vi "运维调试_总磷氨氮.vi"() -> ()   [LabVIEW 2016, in "斯坦道仪器.lvlib"]
uses:
  <vilib>/Platform/TimedLoop/XDataNode/timing_clust.ctl
  <vilib>/Platform/TimedLoop/XDataNode/nitl_modes.ctl
  <vilib>/Platform/TimedLoop/XDataNode/wakeup.ctl
  <vilib>/Utility/miscctls.llb/LVPointTypeDef.ctl
  <vilib>/Platform/TimedLoop/XDataNode/XDataNode.xnode
  <vilib>/Platform/TimedLoop/XDataNode/XDNodeRunTimeDep.lvlib
panel:
  out "固件版本号":string
  in  "参数":T1={"站号"=1, "量程切换"=enum."AUTO", "控制命令"=enum."启动测量", "模式设置"=enum."待机", "测量间隔"=0} {"站号" items=["总磷"=1, "氨氮"=3]}
  out "error out":errorcluster
  in  "同步时间":bool
  in  "数组":string[](array[string])
  in  "备用系数写入":bool
  in  "备用系数读取":bool
  in  "备用系数":T2
  in  "量程切换阈值写入":bool
  in  "量程切换阈值读取":bool
  in  "量程切换阈值":cluster{"阈值":dbl, "标液浓度":dbl}
  in  "参数下拉列表":enum16{"氨氮", "总磷"}(ring)
  in  "量程下拉列表":enum16{"低量程", "高量程"}(ring)
  in  "测量模式下拉列表":enum16{"水样测量", "空白核查", "标样核查", "盲样测试", "加标回收"}(ring)
  in  "公式":cluster{"X^2":dbl, "X":dbl, "b":dbl}
  in  "写公式":bool
  in  "读公式":bool
  in  "精度":dbl=4.0
  in  "样品5 F0":dbl
  in  "样品5 F1":dbl
  in  "样品4 F1":dbl
  in  "样品4 F0":dbl
  in  "样品3 F0":dbl
  in  "样品3 F1":dbl
  in  "样品2 F0":dbl
  in  "样品2 F1":dbl
  in  "样品1 F1":dbl
  in  "样品1 F0":dbl
  in  "method":u16(ring) items=["最小二乘", "最小绝对残差", "Bisquare"]
  in  "模型":enum32{"线性", "多项式"}(ring)
  out "r^2":dbl format="%.7g"
  out "拟合公式":string
  in  "样品2启用":bool
  in  "样品5启用":bool
  in  "样品4启用":bool
  in  "样品3启用":bool
  in  "样品1启用":bool
  in  "标液浓度5":dbl
  out "测量吸光度5":dbl
  in  "标液浓度4":dbl
  out "测量吸光度4":dbl
  in  "标液浓度3":dbl
  out "测量吸光度3":dbl
  in  "标液浓度2":dbl
  out "测量吸光度2":dbl
  out "测量吸光度1":dbl
  in  "标液浓度1":dbl
  out "XY图":cluster{"X Values":dbl[], "Y Values":dbl[]}[](graph)
  in  "返回":bool
  in  "设置":bool
  out "序列号":string="序列号"
  out "氨氮测量数据":T3(xcontrol)
  out "总磷测量数据":T3(xcontrol)
  out "集成报警信息":string
  out "设置值":dbl
  out "定时启动":bool
  out "总磷总氮运行状态":T4(xcontrol)
  in  "停止":bool
  in  "手动启动":bool
  in  "单步测试":bool
  in  "总磷氨氮调试":u16[](xcontrol)
  out "F3":sgl format="%#.6f"
  out "F2":sgl format="%#.6f"
  out "F1":sgl format="%#.6f"
  out "F0":sgl format="%#.6f"
  out "多列列表框":i32(listbox)
  # "COM4"
  # "参数设置"
  # "标液浓度"
  # "F0"
  # "F1"
  # "吸光值显示"
  # "样品一"
  # "辅\n助\n计\n算\n区"
  # "样品二"
  # "样品三"
  # "样品四"
  # "样品五"
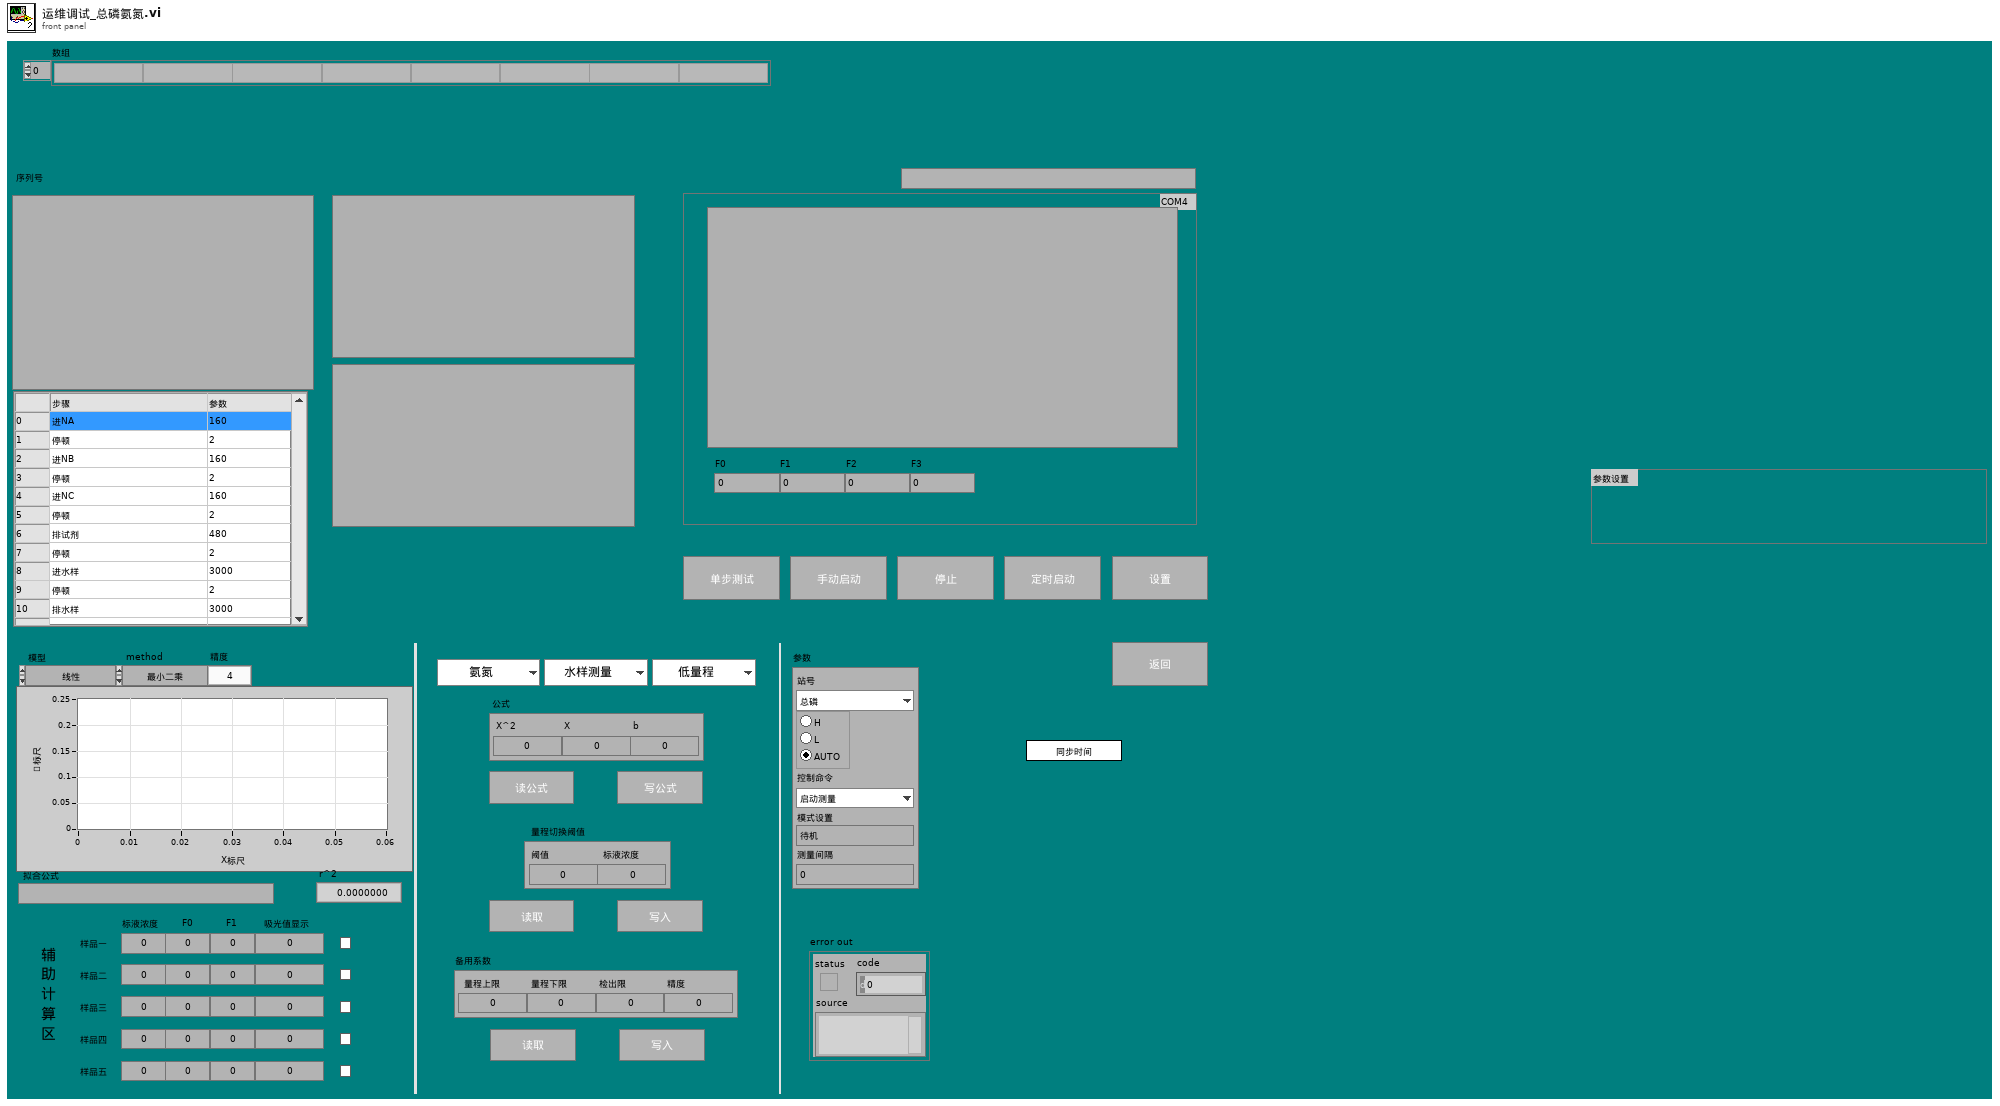
[diagram p1: front panel]
types:
  T1 = cluster{"站号":u16, "量程切换":enum32{"H", "L", "AUTO"}, "控制命令":enum16{"启动测量", "标样核查", "零点核查", "跨度核查", "空白测试", "平行样测试", "加标回收", "空白校准", "标样校准", "初始化（清洗）", "停止测试", "仪器重启", "校时", "模式设置", "测量间隔设置", ""}, "模式设置":enum16{"待机", "连续模式", "周期模式", "定点模式", "受控模式", "手动模式"}, "测量间隔":u16}
  T2 = cluster{"量程上限":dbl, "量程下限":dbl, "检出限":dbl, "精度":dbl}
  T3 = cluster{"flowid":u16, "测量精度":u16, "测量数据区":cluster{"因子编码":u32, "单位":u16, "标样参考值":sgl, "水样数据时间":timestamp, "水样实测值":sgl, "水样数据标识":string, "标样数据时间":timestamp, "标样实测值":sgl, "标样数据标识":string, "空白数据时间":timestamp, "空白实测值":sgl, "空白数据标识":string, "零点核查数据时间":timestamp, "零点核查实测值":sgl, "零点核查数据标识":string, "跨度核查数据时间":timestamp, "跨度核查实测值":sgl, "跨度核查数据标识":string, "加标回收数据时间":timestamp, "加标回收实测值":sgl, "加标回收数据标识":string, "平行样数据时间":timestamp, "平行样实测值":sgl, "平行样数据标识":string}}
  T4 = cluster{"系统时间":timestamp, "工作状态":enum16{"空闲", "水样测试", "标样核查", "零点核查", "跨度核查", "空白测试", "平行样测试", "加标回收", "空白校准", "标样校准", "初始化（清洗）"}, "测量模式":enum16{"待机", "连续模式", "周期模式", "定点模式", "受控模式", "手动模式"}, "告警代码":enum16{"无告警", "缺试剂告警", "缺水样告警", "缺蒸馏水告警", "缺标液告警", "仪表漏液告警", "标定异常告警", "超量程告警", "加热异常", "低试剂预警", "超上限告警", "超下限告警", "仪表内部其他异常", "滴定异常告警", "电极异常告警", "量程切换告警", "参数设置告警", "PH电极电位异常", "电导率电极异常", "浊度光度异常", "溶解氧电极异常", "溶解氧光强异常", "温度异常告警", "PH异常告警", "溶解氧异常告警", "电导率异常告警", "浊度异常告警", "叶绿素异常告警", "藻密度异常告警", "蓝绿藻异常告警", "ORP异常告警", "氨氮异常告警", "清洁刷异常告警", "SD卡异常告警", "蓝牙异常告警", "Wifi异常告警", "流程异常告警"}, "故障代码":enum16{"无故障", "电机故障", "温度故障", "通讯故障", "滴定故障"}, "日志代码":u16, "软件版本":u16, "F0":sgl, "F1":sgl, "F2":sgl, "F3":sgl, "T":sgl, "H":sgl, "id":u16, "flowid":u16, "量程":u16}
  T5 = enum16{"待机", "启动氨氮", "氨氮测量中", "启动总磷", "总磷测量中", "延时"}
  T6 = typedef "LVPointTypeDef.ctl" = cluster{"Horizontal":i16, "Vertical":i16}
  T7 = cluster{"因子编码":u32, "单位":u16, "标样参考值":sgl, "水样数据时间":timestamp, "水样实测值":sgl, "水样数据标识":string, "标样数据时间":timestamp, "标样实测值":sgl, "标样数据标识":string, "空白数据时间":timestamp, "空白实测值":sgl, "空白数据标识":string, "零点核查数据时间":timestamp, "零点核查实测值":sgl, "零点核查数据标识":string, "跨度核查数据时间":timestamp, "跨度核查实测值":sgl, "跨度核查数据标识":string, "加标回收数据时间":timestamp, "加标回收实测值":sgl, "加标回收数据标识":string, "平行样数据时间":timestamp, "平行样实测值":sgl, "平行样数据标识":string}
  T8 = enum16{"空闲", "水样测试", "标样核查", "零点核查", "跨度核查", "空白测试", "平行样测试", "加标回收", "空白校准", "标样校准", "初始化（清洗）"}
  T9 = cluster{"启动模式":enum16{"标液测量", "水样测量", "零液测量", "盲样测量", "加标回收"}, "启动参数":u16, "量程":enum16{"低量程", "高量程"}}
  T10 = cluster{"时间标识":timestamp, "设备":string, "日志信息":string, "流程参数":string}
  T11 = cluster{"时间标识":timestamp, "设备":string, "日志信息":string}
  T12 = enum16{"无告警", "缺试剂告警", "缺水样告警", "缺蒸馏水告警", "缺标液告警", "仪表漏液告警", "标定异常告警", "超量程告警", "加热异常", "低试剂预警", "超上限告警", "超下限告警", "仪表内部其他异常", "滴定异常告警", "电极异常告警", "量程切换告警", "参数设置告警", "PH电极电位异常", "电导率电极异常", "浊度光度异常", "溶解氧电极异常", "溶解氧光强异常", "温度异常告警", "PH异常告警", "溶解氧异常告警", "电导率异常告警", "浊度异常告警", "叶绿素异常告警", "藻密度异常告警", "蓝绿藻异常告警", "ORP异常告警", "氨氮异常告警", "清洁刷异常告警", "SD卡异常告警", "蓝牙异常告警", "Wifi异常告警", "流程异常告警"}
  T13 = typedef "LVRowAndColumnUnsignedTypeDef.ctl" = cluster{"Row":u32, "Column":u32}
  T14 = typedef "XDNodeRunTimeDep.lvlib/timing_clust.ctl" = cluster{"Expected End [f-1]":u64, "Actual End [f-1]":u64, "Finished Late? [f-1]":bool, "Expected End [i-1]":u64, "Actual End [i-1]":u64, "Finished Late? [i-1]":bool, "Expected Start [i]":u64, "Actual Start [i]":u64, "Expected Start [f]":u64, "Actual Start [f]":u64, "Source Name":string, "Structure Name":string, "Period":i64, "Deadline":i64, "Offset":i64, "Start":i64, "Priority":i32, "Timeout":i32, "Mode":T15, "Wakeup Reason":T16, "Error":errorcluster, "Source Type":string, "Secondary Source Type":string, "Global End Time":u64, "Global Start Time":u64, "Frame Duration":u64, "Iteration Duration":u64, "Assigned CPU":i32, "I/O Scan Engine Mode":u32}
  T15 = typedef "XDNodeRunTimeDep.lvlib/nitl_modes.ctl" = enum32{"No Change", "Process missed periods, maintain original phase", "Discard missed periods, maintain original phase", "Process missed periods, ignore original phase", "Discard missed periods, ignore original phase"}
  T16 = typedef "XDNodeRunTimeDep.lvlib/wakeup.ctl" = enum32{"Normal", "Aborted", "Asynchronous wakeup", "Timing source error", "Timed loop error", "Timeout"}
  T17 = cluster{"站号":u16, "量程切换":enum32{"H", "L", "AUTO"}, "控制命令":enum16{"启动测量", "标样核查", "零点核查", "跨度核查", "空白测试", "平行样测试", "加标回收", "空白校准", "标样校准", "初始化（清洗）", "停止测试", "仪器重启", "校时", "模式设置", "测量间隔设置", "盲样测试"}, "模式设置":enum16{"待机", "连续模式", "周期模式", "定点模式", "受控模式", "手动模式"}, "测量间隔":u16}
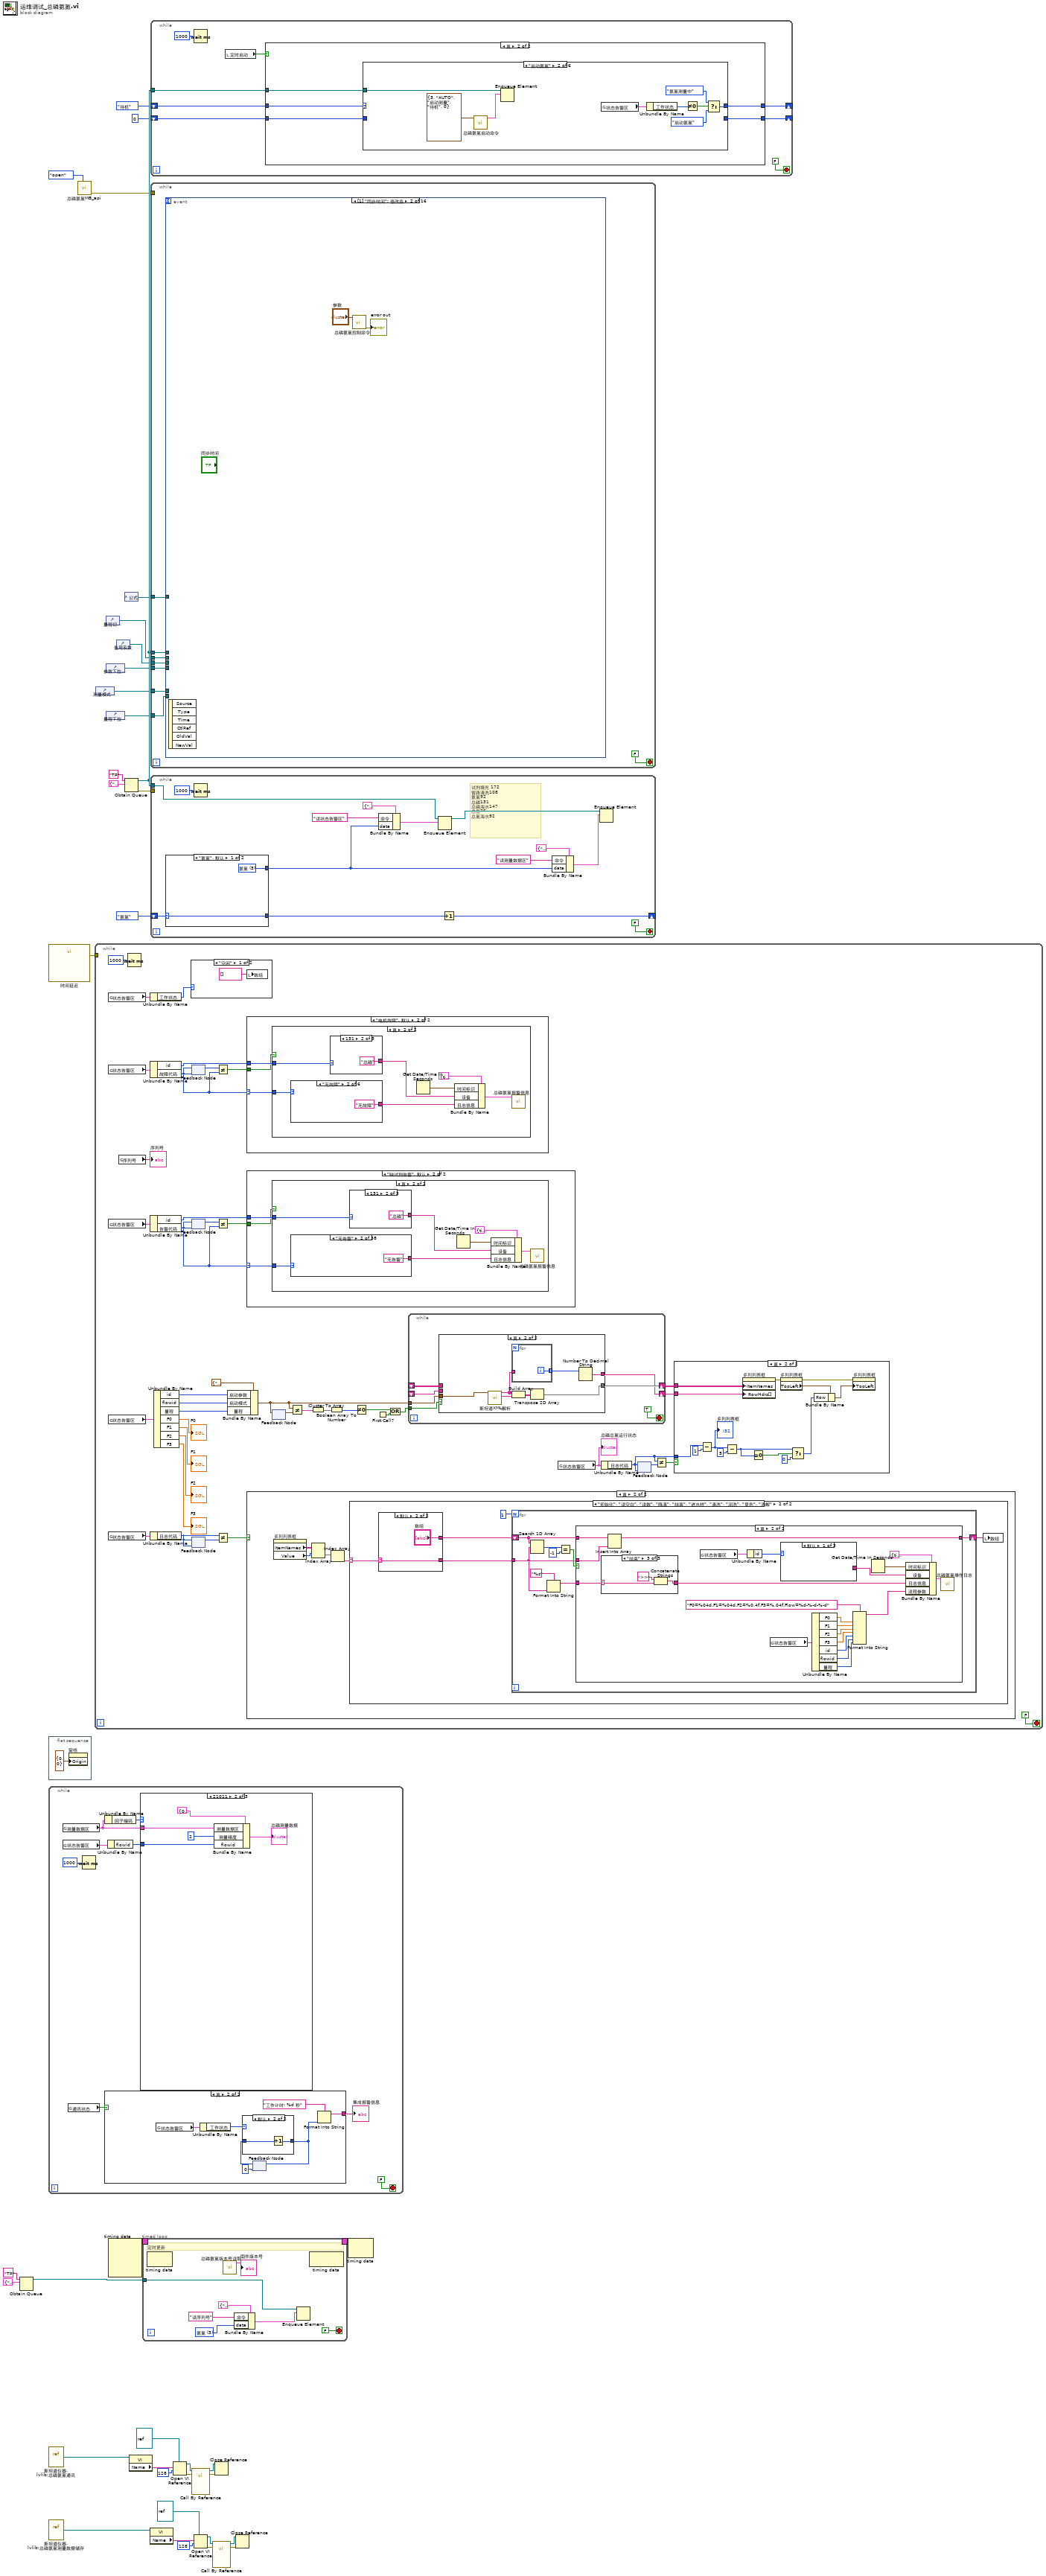
[diagram p0: block diagram]
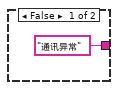
[diagram p2: hidden frame]
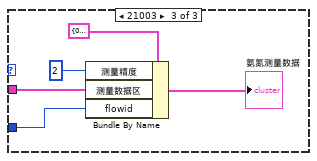
[diagram p5: hidden frame]
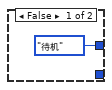
[diagram p6: hidden frame]
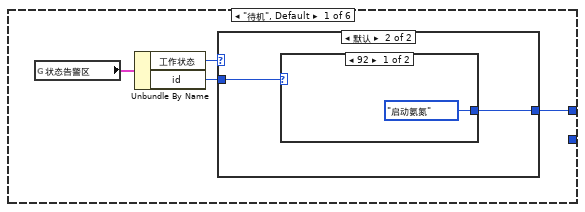
[diagram p7: hidden frame]
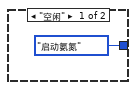
[diagram p8: hidden frame]
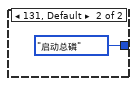
[diagram p9: hidden frame]
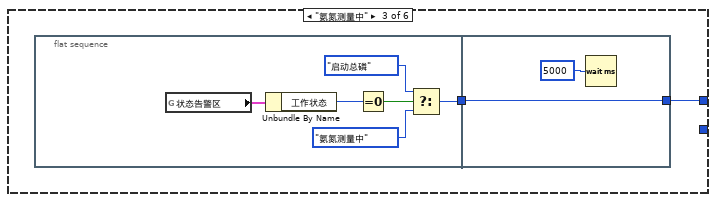
[diagram p10: hidden frame]
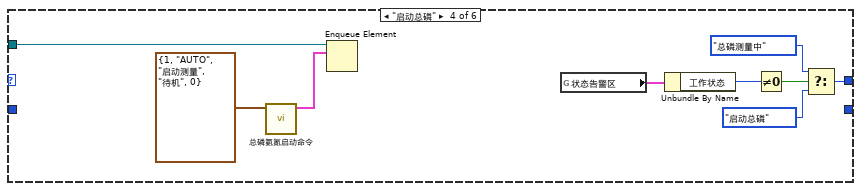
[diagram p11: hidden frame]
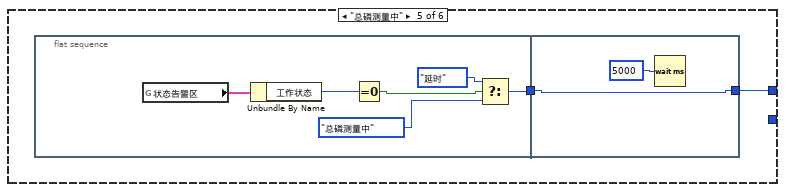
[diagram p12: hidden frame]
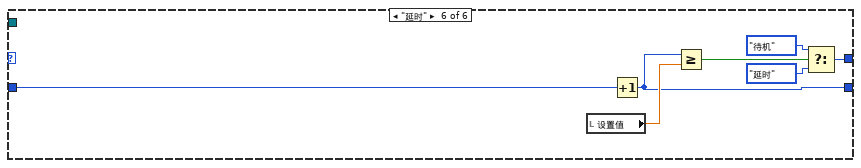
[diagram p13: hidden frame]
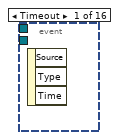
[diagram p14: hidden frame]
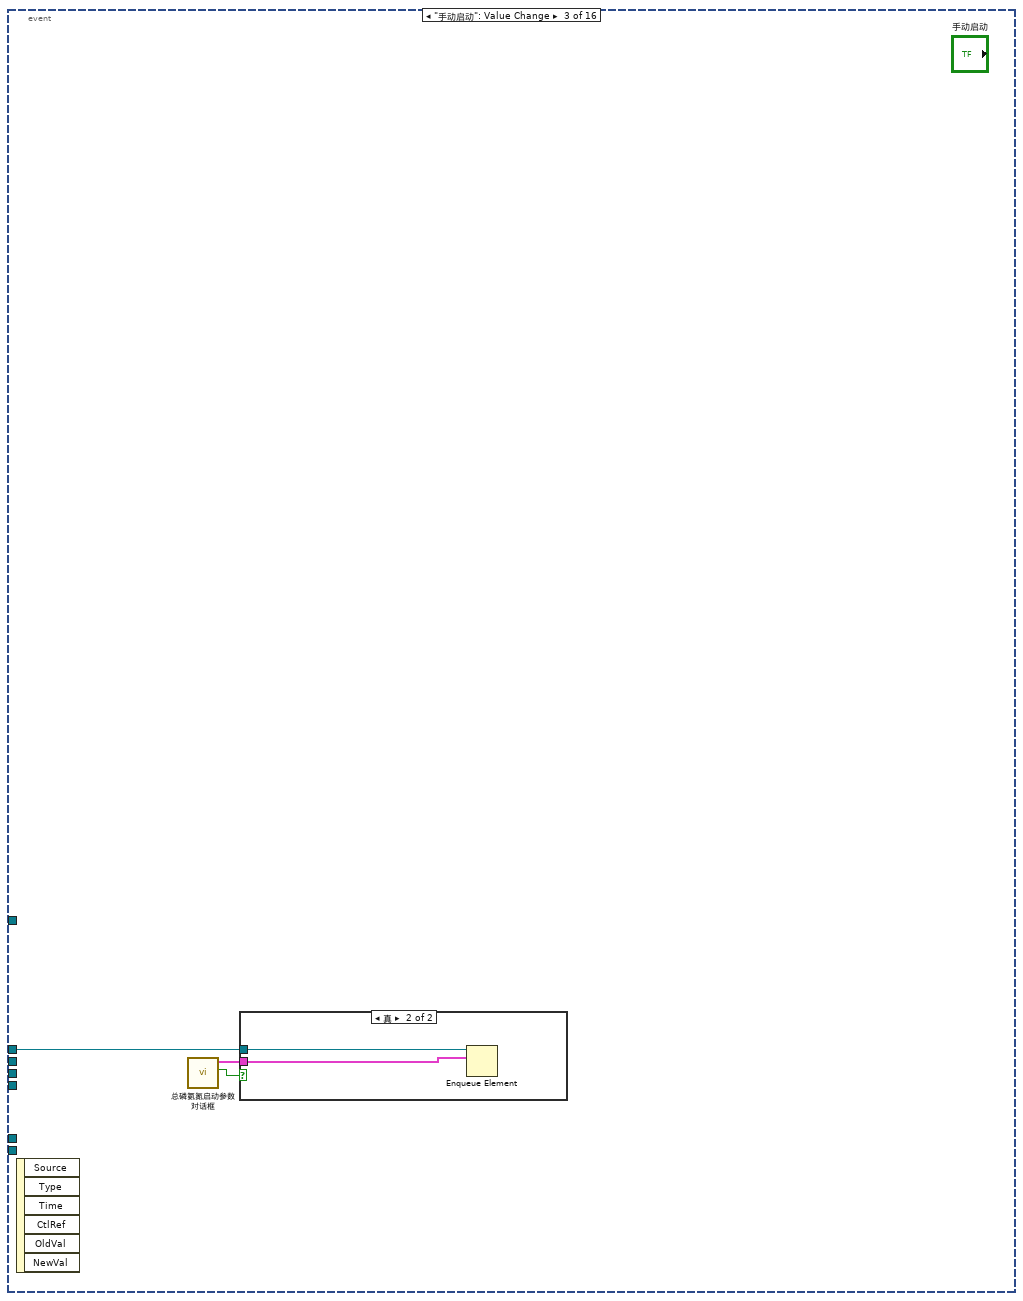
[diagram p15: hidden frame]
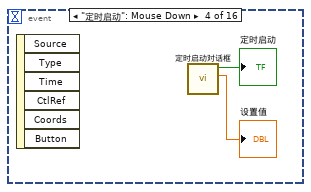
[diagram p17: hidden frame]
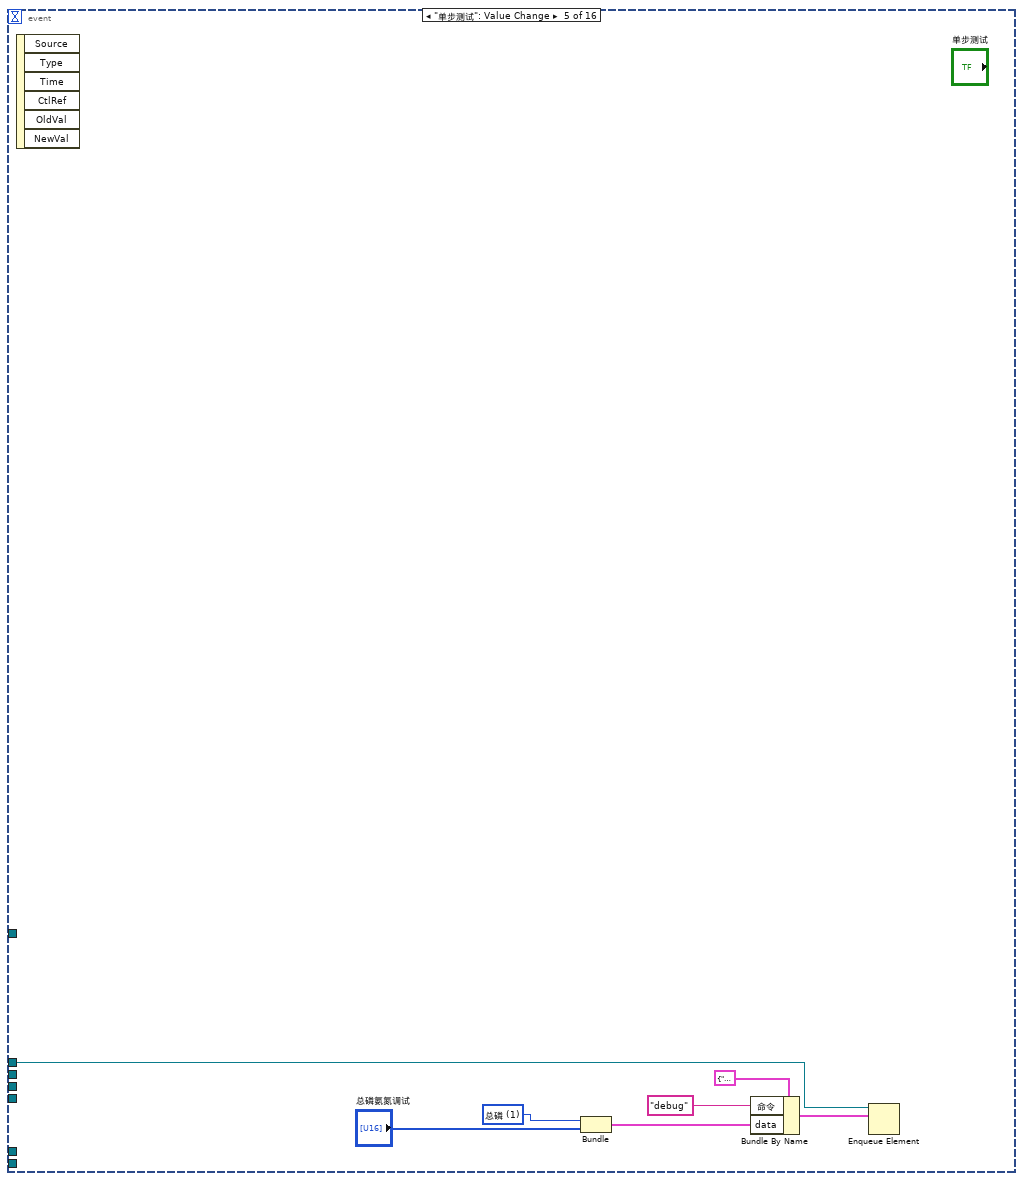
[diagram p18: hidden frame]
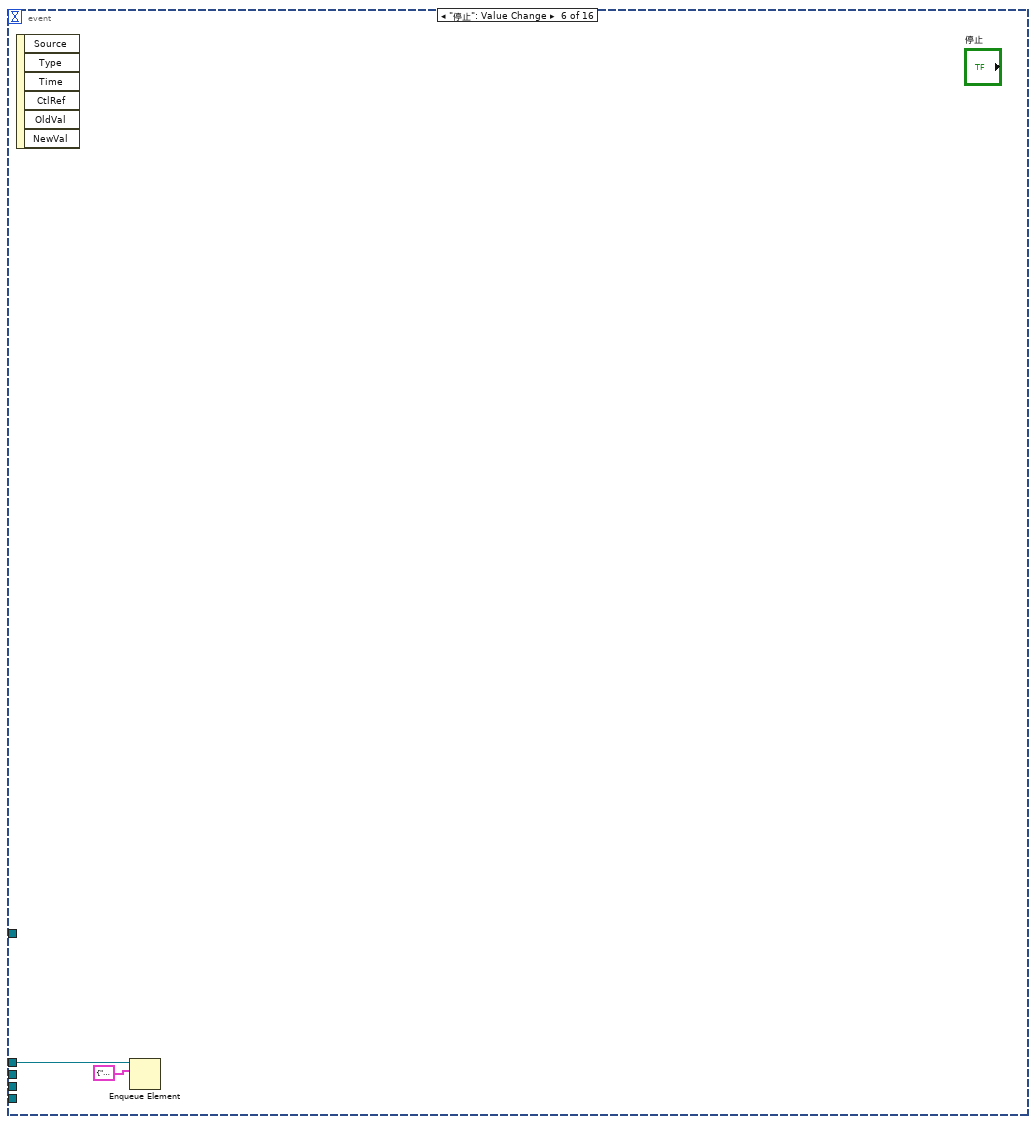
[diagram p19: hidden frame]
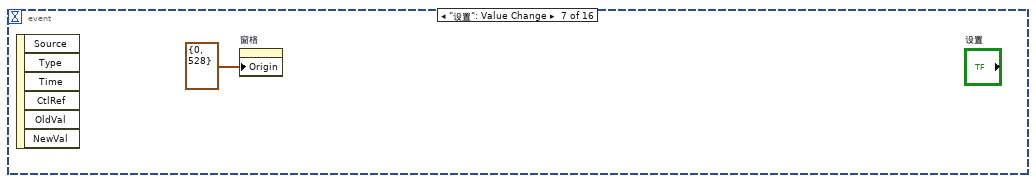
[diagram p20: hidden frame]
diagram:
  n1 = Obtain Queue(name (unnamed)="TP" ("名称（未命名）"), element data type=cluster{"命令":string, "data":variant} {"命令"="", "data"=variant}) -> (queue out=w1:refnum<queue>)  [unwired: 3 in, 2 out]
  n2 = call "时间延迟"() -> ("error out"=w8:errorcluster)  [unwired: 11 in]
  n3 = flat-sequence {
    frame #0 {
      n4 = property on="窗格" class="Pane"("Origin"=T6 {"Horizontal"=0, "Vertical"=0} ("原点")) -> ()  [unwired: 2 in, 2 out]
    }
  }
  n5 = while {
    stop <- FALSE stop-if-true
    n6 = global read "VAR总磷氨氮全局变量.vi" "测量数据区"() -> (w44:T7)
    n7 = global read "VAR总磷氨氮全局变量.vi" "状态告警区"() -> (w40:T4)
    n8 = global read "VAR总磷氨氮全局变量.vi" "通讯状态"() -> (w42:bool)
    n9 = Wait (ms)(milliseconds to wait=u32 1000 ("等待时间（毫秒）")) -> ()  [unwired: 1 out]
    n10 = Unbundle By Name(w44) -> ("因子编码"=w43:u32)
    n11 = case shown="真" w42 {
      tunnel: ["通讯异常" ("集成报警信息") w48] -> w41
      frame False {
      }
      frame True {
        n12 = global read "VAR总磷氨氮全局变量.vi" "状态告警区"() -> (w54:T4)
        n13 = Unbundle By Name(w54) -> ("工作状态"=w53:T8)
        n14 = feedback #1(0) -> (w51:i32)
        n15 = case shown="默认" w53 {
          tunnel: w51 -> [_ w56]
          tunnel: [_ w55] -> w49
          frame "空闲" {
          }
          frame Default {
            n16 = Increment(x=w56) -> (x+1=w55:i32)
          }
        }
        n17 = feedback-in #1(w49) -> ()
        n18 = Format Into String(format string="工作计时: %d 秒" ("格式字符串"), w49) -> (resulting string=w48:string)  [unwired: 2 in, 1 out]
      }
    }
    "集成报警信息" <- w41
    n19 = Unbundle By Name(w40) -> ("flowid"=w39:u16)
    n20 = case shown="21011" w43 {
      tunnel: w44 -> [_ w61 w66]
      tunnel: w39 -> [_ w58 w64]
      frame Default {
      }
      frame 21011 {
        n21 = Bundle By Name(cluster=T3 {"flowid"=0, "测量精度"=0, "测量数据区"={"因子编码"=0, "单位"=0, "标样参考值"=0.0, "水样数据时间"=timestamp(0 s since 1904-01-01), "水样实测值"=0.0, "水样数据标识"="", "标样数据时间"=timestamp(0 s since 1904-01-01), "标样实测值"=0.0, "标样数据标识"="", "空白数据时间"=timestamp(0 s since 1904-01-01), "空白实测值"=0.0, "空白数据标识"="", "零点核查数据时间"=timestamp(0 s since 1904-01-01), "零点核查实测值"=0.0, "零点核查数据标识"="", "跨度核查数据时间"=timestamp(0 s since 1904-01-01), "跨度核查实测值"=0.0, "跨度核查数据标识"="", "加标回收数据时间"=timestamp(0 s since 1904-01-01), "加标回收实测值"=0.0, "加标回收数据标识"="", "平行样数据时间"=timestamp(0 s since 1904-01-01), "平行样实测值"=0.0, "平行样数据标识"=""}} ("氨氮测量数据"), "测量数据区"=w61, "测量精度"=u16 2, "flowid"=w58) -> (→"总磷测量数据":T3)
      }
      frame 21003 {
        n22 = Bundle By Name(cluster=T3 {"flowid"=0, "测量精度"=0, "测量数据区"={"因子编码"=0, "单位"=0, "标样参考值"=0.0, "水样数据时间"=timestamp(0 s since 1904-01-01), "水样实测值"=0.0, "水样数据标识"="", "标样数据时间"=timestamp(0 s since 1904-01-01), "标样实测值"=0.0, "标样数据标识"="", "空白数据时间"=timestamp(0 s since 1904-01-01), "空白实测值"=0.0, "空白数据标识"="", "零点核查数据时间"=timestamp(0 s since 1904-01-01), "零点核查实测值"=0.0, "零点核查数据标识"="", "跨度核查数据时间"=timestamp(0 s since 1904-01-01), "跨度核查实测值"=0.0, "跨度核查数据标识"="", "加标回收数据时间"=timestamp(0 s since 1904-01-01), "加标回收实测值"=0.0, "加标回收数据标识"="", "平行样数据时间"=timestamp(0 s since 1904-01-01), "平行样实测值"=0.0, "平行样数据标识"=""}} ("氨氮测量数据"), "测量精度"=u16 2, "测量数据区"=w66, "flowid"=w64) -> (→"氨氮测量数据":T3)
      }
    }
  }
  n23 = vi-ref "斯坦道仪器.lvlib:总磷氨氮通讯.vi"() -> (w31:refnum<vi>)
  n24 = vi-ref "斯坦道仪器.lvlib:总磷氨氮测量数据储存.vi"() -> (w23:refnum<vi>)
  n25 = call "总磷氨氮MB_api.vi"("STEP"=enum16{"open", "read", "write", "close"}."open") -> ("error out"=w7:errorcluster)  [unwired: 8 in, 2 out]
  n26 = while {
    tunnel: w8 -> [_]
    stop <- FALSE stop-if-true
    n27 = global read "VAR总磷氨氮全局变量.vi" "状态告警区"() -> (w72:T4)
    n28 = global read "VAR总磷氨氮全局变量.vi" "状态告警区"() -> (w78:T4)
    n29 = global read "VAR总磷氨氮全局变量.vi" "状态告警区"() -> (w83:T4)
    n30 = global read "VAR总磷氨氮全局变量.vi" "状态告警区"() -> (w95:T4)
    n31 = global read "VAR总磷氨氮全局变量.vi" "状态告警区"() -> (w69:T4)
    n32 = global read "VAR总磷氨氮全局变量.vi" "序列号"() -> (→"序列号":string)
    n33 = Wait (ms)(milliseconds to wait=u32 1000 ("等待时间（毫秒）")) -> ()  [unwired: 1 out]
    n34 = Unbundle By Name(w72) -> ("工作状态"=w71:T8)
    n35 = Unbundle By Name(w78) -> ("id"=w77:u16, "故障代码"=w74:enum16{"无故障", "电机故障", "温度故障", "通讯故障", "滴定故障"})
    n36 = Unbundle By Name(w83) -> ("id"=w82:u16, "告警代码"=w79:T12)
    n37 = Unbundle By Name(w69) -> ("日志代码"=w68:u16)
    n38 = Unbundle By Name(w95) -> ("id"=w92:u16, "flowid"=w94:u16, "量程"=w93:u16, "F0"=→"F0":sgl, "F1"=→"F1":sgl, "F2"=→"F2":sgl, "F3"=→"F3":sgl)
    n39 = case shown="\"空闲\"" w71 {
      frame "空闲" {
        n40 = local write "数组"(string[] [] ("数组")) -> ()
      }
      frame "水样测试", Default {
      }
    }
    n41 = feedback #2(w74) -> (w75:enum16{"无故障", "电机故障", "温度故障", "通讯故障", "滴定故障"})
    n42 = feedback-in #2(w74) -> ()
    n43 = feedback #3(w79) -> (w80:T12)
    n44 = feedback-in #3(w79) -> ()
    n45 = feedback #4(w68) -> (w70:u16)
    n46 = feedback-in #4(w68) -> ()
    n47 = Not Equal?(x=w75, y=w74) -> (x != y?=w76:bool)
    n48 = Not Equal?(x=w80, y=w79) -> (x != y?=w81:bool)
    n49 = Not Equal?(x=w68, y=w70) -> (x != y?=w67:bool)
    n50 = Bundle By Name(cluster=T9 {"启动模式"=enum."加标回收", "启动参数"=1, "量程"=enum."低量程"} ("参数簇"), "启动参数"=w92, "启动模式"=w94, "量程"=w93) -> (w85:T9)
    n51 = case shown="\"电机故障\", 默认" w74 {
      selector: w74 -> [_ w163]
      tunnel: w77 -> [_ w164]
      tunnel: w76 -> [_ w162]
      frame "无故障" {
      }
      frame "电机故障", Default {
        n52 = case shown="真" w162 {
          tunnel: w164 -> [_ w171]
          tunnel: w163 -> [_ w166]
          frame False {
          }
          frame True {
            n53 = case shown="\"无故障\"" w166 {
              selector: w166 -> [w173 _ _ _ _ _]
              tunnel: [w172 "无故障" "电机故障" "温度故障" "通讯故障" "滴定故障"] -> w165
              frame Default {
                n54 = Format Into String(format string="%d" ("格式字符串"), initial string="未知" ("工作状态"), w173) -> (resulting string=w172:string)  [unwired: 1 in, 1 out]
              }
              frame "无故障" {
              }
              frame "电机故障" {
              }
              frame "温度故障" {
              }
              frame "通讯故障" {
              }
              frame "滴定故障" {
              }
            }
            n55 = case shown="131" w171 {
              tunnel: [_ "总磷" ("table输入") "氨氮" ("table输入")] -> w167
              frame Default {
              }
              frame 131 {
              }
              frame 92 {
              }
            }
            n56 = Get Date/Time In Seconds() -> (seconds since 1Jan1904=w168:timestamp)
            n57 = Bundle By Name(cluster=T11 {"时间标识"=timestamp(0 s since 1904-01-01), "设备"="", "日志信息"=""} ("data in"), "时间标识"=w168, "设备"=w167, "日志信息"=w165) -> (w169:T11)
            n58 = call "总磷氨氮报警信息.vi"("data in"=w169) -> ()  [unwired: 11 in]
          }
        }
      }
    }
    n59 = case shown="\"缺试剂告警\", 默认" w79 {
      selector: w79 -> [_ w184]
      tunnel: w82 -> [_ w185]
      tunnel: w81 -> [_ w183]
      frame "无告警" {
      }
      frame "缺试剂告警", Default {
        n60 = case shown="真" w183 {
          tunnel: w185 -> [_ w192]
          tunnel: w184 -> [_ w186]
          frame False {
          }
          frame True {
            n61 = case shown="\"无告警\"" w186 {
              selector: w186 -> [w194 _ _ _ _ _ _ _ _ _ _ _ _ _ _ _ _ _ _ _ _ _ _ _ _ _ _ _ _ _ _ _ _ _ _ _ _ _]
              tunnel: [w193 "无告警" "缺试剂告警" "缺水样告警" "缺蒸馏水告警" "缺标液告警" "仪表漏液告警" "标定异常告警" "超量程告警" "加热异常" "低试剂预警" "超上限告警" "超下限告警" "仪表内部其他异常" "滴定异常告警" "电极异常告警" "量程切换告警" "参数设置告警" "PH电极电位异常" "电导率电极异常" "浊度光度异常" "溶解氧电极异常" "溶解氧光强异常" "温度异常告警" "PH异常告警" "溶解氧异常告警" "电导率异常告警" "浊度异常告警" "叶绿素异常告警" "藻密度异常告警" "蓝绿藻异常告警" "ORP异常告警" "氨氮异常告警" "清洁刷异常告警" "SD卡异常告警" "蓝牙异常告警" "WiFi异常告警" "流程异常告警"] -> w187
              frame Default {
                n62 = Format Into String(format string="%d" ("格式字符串"), initial string="未知" ("工作状态"), w194) -> (resulting string=w193:string)  [unwired: 1 in, 1 out]
              }
              frame "无告警" {
              }
              frame "缺试剂告警" {
              }
              frame "缺水样告警" {
              }
              frame "缺蒸馏水告警" {
              }
              frame "缺标液告警" {
              }
              frame "仪表漏液告警" {
              }
              frame "标定异常告警" {
              }
              frame "超量程告警" {
              }
              frame "加热异常" {
              }
              frame "低试剂预警" {
              }
              frame "超上限告警" {
              }
              frame "超下限告警" {
              }
              frame "仪表内部其他异常" {
              }
              frame "滴定异常告警" {
              }
              frame "电极异常告警" {
              }
              frame "量程切换告警" {
              }
              frame "参数设置告警" {
              }
              frame "PH电极电位异常" {
              }
              frame "电导率电极异常" {
              }
              frame "浊度光度异常" {
              }
              frame "溶解氧电极异常" {
              }
              frame "溶解氧光强异常" {
              }
              frame "温度异常告警" {
              }
              frame "PH异常告警" {
              }
              frame "溶解氧异常告警" {
              }
              frame "电导率异常告警" {
              }
              frame "浊度异常告警" {
              }
              frame "叶绿素异常告警" {
              }
              frame "藻密度异常告警" {
              }
              frame "蓝绿藻异常告警" {
              }
              frame "ORP异常告警" {
              }
              frame "氨氮异常告警" {
              }
              frame "清洁刷异常告警" {
              }
              frame "SD卡异常告警" {
              }
              frame "蓝牙异常告警" {
              }
              frame "Wifi异常告警" {
              }
              frame "流程异常告警" {
              }
            }
            n63 = case shown="131" w192 {
              tunnel: [_ "总磷" ("table输入") "氨氮" ("table输入")] -> w188
              frame Default {
              }
              frame 131 {
              }
              frame 92 {
              }
            }
            n64 = Get Date/Time In Seconds() -> (seconds since 1Jan1904=w189:timestamp)
            n65 = Bundle By Name(cluster=T11 {"时间标识"=timestamp(0 s since 1904-01-01), "设备"="", "日志信息"=""} ("data in"), "时间标识"=w189, "设备"=w188, "日志信息"=w187) -> (w190:T11)
            n66 = call "总磷氨氮报警信息.vi"("data in"=w190) -> ()  [unwired: 11 in]
          }
        }
      }
    }
    n67 = case shown="真" w67 {
      frame False {
      }
      frame True {
        n68 = property on="多列列表框" class="MCListbox (严格)"() -> ("ItemNames"=w112:string[][], "Value"=w113:i32)  [unwired: 2 in, 2 out]
        n69 = Index Array(array=w112, index (row)=w113) -> (element=w111:string[])  [unwired: 1 in]
        n70 = Index Array(array=w111) -> (element=w110:string)  [unwired: 1 in]
        n71 = case shown="\"初始化\", \"读空白\", \"读数\", \"降温\", \"结束\", \"进水样\", \"清洗\", \"润洗\", \"显色\", \"消解\"" w110 {
          selector: w110 -> [_ w116]
          frame Default {
          }
          frame "初始化", "读空白", "读数", "降温", "结束", "进水样", "清洗", "润洗", "显色", "消解" {
            n72 = case shown="默认" w116 {
              selector: w116 -> [w120 w122]
              tunnel: [w120 w122] -> w115
              tunnel: [string[] [] ("数组") "数组"] -> w114
              frame "读数" {
              }
              frame Default {
              }
            }
            n73 = for {
              N: 1 -> [_]
              tunnel: w115 -> [w124]
              shift-right: [w123] -> w117
              shift-left: w114 -> [w125]
              n74 = Search 1D Array(1D array=w125, element=w124) -> (index of element=w128:i32)  [unwired: 1 in]
              n75 = Format Into String(format string="%s" ("格式字符串"), w124) -> (resulting string=w129:string)  [unwired: 2 in, 1 out]
              n76 = Equal?(x=w128, y=-1) -> (x = y?=w126:bool)
              n77 = case shown="真" w126 {
                tunnel: w129 -> [_ w133]
                tunnel: w125 -> [w131 w137]
                tunnel: w124 -> [_ w136]
                tunnel: [w131 w135] -> w123
                frame False {
                }
                frame True {
                  n78 = case shown="\"结束\"" w133 {
                    selector: w133 -> [w153 w156 w159]
                    tunnel: [w153 w155 w158] -> w132
                    frame Default {
                    }
                    frame "初始化" {
                      n79 = Concatenate Strings("<<" ("字符串"), w156) -> (w155:string)
                    }
                    frame "结束" {
                      n80 = Concatenate Strings(">>" ("字符串"), w159) -> (w158:string)
                    }
                  }
                  n81 = Insert Into Array(array=w137, new element=w136) -> (w135:string[])  [unwired: 1 in]
                  n82 = global read "VAR总磷氨氮全局变量.vi" "状态告警区"() -> (w152:T4)
                  n83 = Unbundle By Name(w152) -> ("id"=w151:u16)
                  n84 = global read "VAR总磷氨氮全局变量.vi" "状态告警区"() -> (w147:T4)
                  n85 = case shown="默认" w151 {
                    tunnel: [_ "总磷" ("table输入") "氨氮" ("table输入")] -> w149
                    frame Default {
                    }
                    frame 131 {
                    }
                    frame 92 {
                    }
                  }
                  n86 = Unbundle By Name(w147) -> ("F0"=w144:sgl, "F1"=w143:sgl, "F2"=w142:sgl, "F3"=w141:sgl, "id"=w140:u16, "flowid"=w139:u16, "量程"=w138:u16)
                  n87 = Format Into String(format string="F0=%04d,F1=%04d,F2=%0.4f,F3=%.04f,Flow=%d-%-d-%-d" ("格式字符串"), w144, w143, w142, w141, w140, w139, w138) -> (resulting string=w145:string)  [unwired: 2 in, 1 out]
                  n88 = Get Date/Time In Seconds() -> (seconds since 1Jan1904=w148:timestamp)
                  n89 = Bundle By Name(cluster=T10 {"时间标识"=timestamp(0 s since 1904-01-01), "设备"="", "日志信息"="", "流程参数"=""} ("data in"), "时间标识"=w148, "设备"=w149, "日志信息"=w132, "流程参数"=w145) -> (w150:T10)
                  n90 = call "总磷氨氮操作日志.vi"("data in"=w150) -> ()  [unwired: 11 in]
                }
              }
            }
            n91 = local write "数组"(w117) -> ()
          }
        }
      }
    }
    n92 = feedback #5() -> (w101:T9)  [unwired: 1 in]
    n93 = feedback-in #5(w85) -> ()
    n94 = Not Equal?(x=w85, y=w101) -> (x != y?=w102:cluster{"启动模式":bool, "启动参数":bool, "量程":bool})
    n95 = Cluster To Array(cluster=w102) -> (array=w103:bool[])
    n96 = Boolean Array To Number(Boolean array=w103) -> (number=w104:u32)
    n97 = Not Equal To 0?(x=w104) -> (x != 0?=w97:bool)
    n98 = First Call?() -> (First Call?: T/F=w98:bool)
    n99 = Or(x=w97, y=w98) -> (x .or. y?=w96:bool)
    n100 = while {
      tunnel: w96 -> [w242]
      tunnel: w85 -> [w241]
      shift-right: [w240] -> w100
      shift-left: _ -> [w236]
      shift-right: [w239] -> w99
      shift-left: _ -> [w237]
      stop <- TRUE stop-if-true
      n101 = case shown="真" w242 {
        tunnel: [w244 w251] -> w239
        tunnel: [w243 w250] -> w240
        tunnel: w241 -> [_ w245]
        tunnel: w237 -> [w244 _]
        tunnel: w236 -> [w243 _]
        frame False {
        }
        frame True {
          n102 = call "斯坦道XML解析.vi"("参数簇"=w245) -> ("步骤时间"=w246:string[], "步骤名"=w248:string[])  [unwired: 9 in]
          n103 = for {
            tunnel: w248 -> [_] mode=indexing
            tunnel: [w252] -> w249 mode=indexing
            i -> [w252]
          }
          n104 = Build Array(w248, w246) -> (w247:string[][])
          n105 = Transpose 2D Array(2D array=w247) -> (transposed array=w250:string[][])
          n106 = Number To Decimal String(number=w249) -> (decimal integer string=w251:string[])  [unwired: 1 in]
        }
      }
    }
    n107 = global read "VAR总磷氨氮全局变量.vi" "状态告警区"() -> (w86:T4)
    "总磷总氮运行状态" <- w86
    n108 = Unbundle By Name(w86) -> ("日志代码"=w73:u16)
    n109 = feedback-in #6(w73) -> ()
    n110 = feedback #6(w73) -> (w106:u16)
    n111 = Not Equal?(x=w73, y=w106) -> (x != y?=w105:bool)
    n112 = case shown="真" w105 {
      tunnel: w73 -> [_ w255]
      tunnel: w100 -> [_ w262]
      tunnel: w99 -> [_ w261]
      frame False {
      }
      frame True {
        n113 = Subtract(x=w255, y=1) -> (x-y=w253:i32)
        "多列列表框" <- w253
        n114 = Subtract(x=w253, y=5) -> (x-y=w257:i32)
        n115 = property on="多列列表框" class="MCListbox (严格)"("ItemNames"=w262, "RowHdrs[]"=w261) -> (error out=w263:errorcluster)  [unwired: 2 in, 1 out]
        n116 = Greater Or Equal To 0?(x=w257) -> (x >= 0?=w256:bool)
        n117 = property on="多列列表框" class="MCListbox (严格)"(error in=w263) -> (error out=w264:errorcluster, "TopLeft"=w265:T13)  [unwired: 1 in, 1 out]
        n118 = Select(t=w257, s=w256, f=0) -> (s? t:f=w258:i32)
        n119 = Bundle By Name(cluster=w265, "Row"=w258) -> (w266:T13)
        n120 = property on="多列列表框" class="MCListbox (严格)"(error in=w264, "TopLeft"=w266) -> ()  [unwired: 1 in, 2 out]
      }
    }
  }
  n121 = control-ref of="测量模式下拉列表"() -> (w12:refnum<vi>)
  n122 = control-ref of="量程切换阈值"() -> (w10:refnum<vi>)
  n123 = control-ref of="参数下拉列表"() -> (w13:refnum<vi>)
  n124 = control-ref of="量程下拉列表"() -> (w14:refnum<vi>)
  n125 = node-c288() -> (w5:T14)  [unwired: 4 in]
  n126 = control-ref of="备用系数"() -> (w9:refnum<vi>)
  n127 = control-ref of="公式"() -> (w11:refnum<vi>)
  n128 = Obtain Queue(name (unnamed)="TP" ("名称（未命名）"), element data type=cluster{"命令":string, "data":variant} {"命令"="", "data"=variant}) -> (queue out=w34:refnum<queue>, error out=w35:errorcluster)  [unwired: 3 in, 1 out]
  n129 = property class="VI"(reference=w31) -> ("Name"=w30:string)  [unwired: 1 in, 2 out]
  n130 = timed-loop {
    timing: w5 -> [_]
    timing-out: [_] -> w4
    tunnel: w1 -> [w269]
    stop <- FALSE stop-if-true
    w270 = u16 3 items=["总磷"=1, "氨氮"=3] ("站号")
    # "定时更新"
    n131 = node-c288() -> ()  [unwired: 1 in, 1 out]
    n132 = call "总磷氨氮版本号读取.vi"() -> ("固件版本号"=→"固件版本号":string)  [unwired: 11 in]
    n133 = Bundle By Name(cluster=cluster{"命令":string, "data":variant} {"命令"="", "data"=variant} ("元素"), "命令"="读序列号", "data"=w270) -> (w268:cluster{"命令":string, "data":variant})
    n134 = Enqueue Element(queue=w269, element=w268) -> ()  [unwired: 2 in, 3 out]
    n135 = node-c288() -> ()  [unwired: 1 in, 1 out]
  }
  n136 = property class="VI"(reference=w23) -> ("Name"=w16:string)  [unwired: 1 in, 2 out]
  n137 = while {
    tunnel: w34 -> [w278]
    shift-right: [w279] -> _
    shift-left: T5."待机" -> [w280]
    shift-right: [w276] -> _
    shift-left: u32 0 ("等待时间（毫秒）") -> [w277]
    stop <- FALSE stop-if-true
    n138 = Wait (ms)(milliseconds to wait=u32 1000 ("等待时间（毫秒）")) -> ()  [unwired: 1 out]
    n139 = local read "定时启动"() -> (w281:bool)
    n140 = case shown="真" w281 {
      tunnel: w280 -> [_ w289]
      tunnel: [T5."待机" w288] -> w279
      tunnel: w278 -> [_ w287]
      tunnel: w277 -> [_ w286]
      tunnel: [_ w285] -> w276
      frame False {
      }
      frame True {
        n141 = case shown="\"启动氨氮\"" w289 {
          tunnel: [w290 w302 w309 w320 w328 w340] -> w288
          tunnel: w287 -> [_ w307 _ w326 _ _]
          tunnel: w286 -> [_ _ _ _ _ w343]
          tunnel: [_ _ _ _ _ w339] -> w285
          frame "待机", Default {
            n142 = global read "VAR总磷氨氮全局变量.vi" "状态告警区"() -> (w293:T4)
            n143 = Unbundle By Name(w293) -> ("工作状态"=w291:T8, "id"=w292:u16)
            n144 = case shown="默认" w291 {
              tunnel: w292 -> [_ w296]
              tunnel: [T5."启动氨氮" w295] -> w290
              frame "空闲" {
              }
              frame Default {
                n145 = case shown="92" w296 {
                  tunnel: [T5."启动氨氮" T5."启动总磷"] -> w295
                  frame 92 {
                  }
                  frame 131, Default {
                  }
                }
              }
            }
          }
          frame "启动氨氮" {
            n146 = call "总磷氨氮启动命令.vi"("参数"=T17 {"站号"=3, "量程切换"=enum."AUTO", "控制命令"=enum."启动测量", "模式设置"=enum."待机", "测量间隔"=0}) -> ("启动命令"=w300:cluster{"命令":string, "data":variant})  [unwired: 10 in]
            n147 = Enqueue Element(queue=w307, element=w300) -> ()  [unwired: 2 in, 3 out]
            n148 = global read "VAR总磷氨氮全局变量.vi" "状态告警区"() -> (w306:T4)
            n149 = Unbundle By Name(w306) -> ("工作状态"=w305:T8)
            n150 = Not Equal To 0?(x=w305) -> (x != 0?=w304:bool)
            n151 = Select(t=T5."氨氮测量中", s=w304, f=T5."启动氨氮") -> (s? t:f=w302:T5)
          }
          frame "氨氮测量中" {
            n152 = flat-sequence {
              tunnel: [w313] -> w308
              tunnel: [w317] -> w309
              tunnel: w308 -> [w317]
              frame #0 {
                n153 = global read "VAR总磷氨氮全局变量.vi" "状态告警区"() -> (w314:T4)
                n154 = Unbundle By Name(w314) -> ("工作状态"=w315:T8)
                n155 = Equal To 0?(x=w315) -> (x = 0?=w310:bool)
                n156 = Select(t=T5."启动总磷", s=w310, f=T5."氨氮测量中") -> (s? t:f=w313:T5)
              }
              frame #1 {
                n157 = Wait (ms)(milliseconds to wait=u32 5000 ("等待时间（毫秒）")) -> ()  [unwired: 1 out]
              }
            }
          }
          frame "启动总磷" {
            n158 = call "总磷氨氮启动命令.vi"("参数"=T17 {"站号"=1, "量程切换"=enum."AUTO", "控制命令"=enum."启动测量", "模式设置"=enum."待机", "测量间隔"=0}) -> ("启动命令"=w319:cluster{"命令":string, "data":variant})  [unwired: 10 in]
            n159 = Enqueue Element(queue=w326, element=w319) -> ()  [unwired: 2 in, 3 out]
            n160 = global read "VAR总磷氨氮全局变量.vi" "状态告警区"() -> (w321:T4)
            n161 = Unbundle By Name(w321) -> ("工作状态"=w322:T8)
            n162 = Not Equal To 0?(x=w322) -> (x != 0?=w323:bool)
            n163 = Select(t=T5."总磷测量中", s=w323, f=T5."启动总磷") -> (s? t:f=w320:T5)
          }
          frame "总磷测量中" {
            n164 = flat-sequence {
              tunnel: [w330] -> w327
              tunnel: [w336] -> w328
              tunnel: w327 -> [w336]
              frame #0 {
                n165 = global read "VAR总磷氨氮全局变量.vi" "状态告警区"() -> (w333:T4)
                n166 = Unbundle By Name(w333) -> ("工作状态"=w334:T8)
                n167 = Equal To 0?(x=w334) -> (x = 0?=w329:bool)
                n168 = Select(t=T5."延时", s=w329, f=T5."总磷测量中") -> (s? t:f=w330:T5)
              }
              frame #1 {
                n169 = Wait (ms)(milliseconds to wait=u32 5000 ("等待时间（毫秒）")) -> ()  [unwired: 1 out]
              }
            }
          }
          frame "延时" {
            n170 = local read "设置值"() -> (w342:dbl)
            n171 = Increment(x=w343) -> (x+1=w339:u32)
            n172 = Greater Or Equal?(x=w339, y=w342) -> (x >= y?=w341:bool)
            n173 = Select(t=T5."待机", s=w341, f=T5."延时") -> (s? t:f=w340:T5)
          }
        }
      }
    }
  }
  n174 = while {
    tunnel: w34 -> [w350]
    tunnel: w14 -> [w349]
    tunnel: w13 -> [w348]
    tunnel: w12 -> [w347]
    tunnel: w11 -> [w346]
    tunnel: w10 -> [w345]
    tunnel: w9 -> [w344]
    tunnel: w7 -> [_]
    stop <- FALSE stop-if-true
    n175 = event shown="[1] \"同步时间\": 值改变" {
      selector: _ -> [_ _ _ _ _ _ _ _ _ _ _ _ _ _ _ _]
      dyn-events: _ -> [_ _ _ _ _ _ _ _ _ _ _ _ _ _ _ _]
      timeout: _ -> [_ _ _ _ _ _ _ _ _ _ _ _ _ _ _ _]
      tunnel: w350 -> [_ _ w356 _ w367 w369 _ _ _ _ _ _ _ _ _ _]
      tunnel: w349 -> [_ _ _ _ _ _ _ _ _ _ w422 _ w442 w451 _ _]
      tunnel: w348 -> [_ _ _ _ _ _ _ _ _ _ w420 _ w440 w453 w461 w468]
      tunnel: w347 -> [_ _ _ _ _ _ _ _ _ _ w421 _ w441 w452 _ _]
      tunnel: w346 -> [_ _ _ _ _ _ _ _ _ _ w416 _ _ _ _ _]
      tunnel: w345 -> [_ _ _ _ _ _ _ _ _ _ _ _ w436 _ _ _]
      tunnel: w344 -> [_ _ _ _ _ _ _ _ _ _ _ _ _ _ w459 _]
      event Timeout {
        n176 = event-data() -> ()  [unwired: 1 in, 3 out]
      }
      event "同步时间": Value Change {
        n177 = event-data() -> ()  [unwired: 1 in, 6 out]
        n178 = call "总磷氨氮控制命令.vi"("参数"="参数") -> ("error out"=→"error out":errorcluster)  [unwired: 10 in]
      }
      event "手动启动": Value Change {
        n179 = event-data() -> ()  [unwired: 1 in, 6 out]
        n180 = call "总磷氨氮启动参数对话框.vi"() -> ("确认"=w354:bool, "元素"=w355:cluster{"命令":string, "data":variant})  [unwired: 10 in]
        n181 = case shown="真" w354 {
          tunnel: w356 -> [_ w358]
          tunnel: w355 -> [_ w357]
          frame False {
          }
          frame True {
            n182 = Enqueue Element(queue=w358, element=w357) -> ()  [unwired: 2 in, 3 out]
          }
        }
      }
      event "定时启动": Mouse Down {
        n183 = event-data() -> ()  [unwired: 1 in, 6 out]
        n184 = call "定时启动对话框.vi"() -> ("设置值"=→"设置值":dbl, "确定输出"=→"定时启动":bool)  [unwired: 10 in]
      }
      event "单步测试": Value Change {
        w362 = u16 1 items=["总磷"=1, "氨氮"=3] ("站号")
        n185 = event-data() -> ()  [unwired: 1 in, 6 out]
        n186 = Bundle("站号"=w362, "总磷氨氮调试"="总磷氨氮调试") -> (w361:cluster{"站号":u16, "总磷氨氮调试":u16[]})  [unwired: 1 in]
        n187 = Bundle By Name(cluster=cluster{"命令":string, "data":variant} {"命令"="", "data"=variant} ("元素"), "命令"="debug", "data"=w361) -> (w364:cluster{"命令":string, "data":variant})
        n188 = Enqueue Element(queue=w367, element=w364) -> ()  [unwired: 2 in, 3 out]
      }
      event "停止": Value Change {
        n189 = event-data() -> ()  [unwired: 1 in, 6 out]
        n190 = Enqueue Element(queue=w369, element=cluster{"命令":string, "data":variant} {"命令"="启动", "data"=variant(cluster{"站号":u16, "控制命令输出":u16[]} {"站号"=1, "控制命令输出"=[2816]})} ("元素")) -> ()  [unwired: 2 in, 3 out]
      }
      event "设置": Value Change {
        n191 = event-data() -> ()  [unwired: 1 in, 6 out]
        n192 = property on="窗格" class="Pane"("Origin"=T6 {"Horizontal"=0, "Vertical"=528} ("原点")) -> ()  [unwired: 2 in, 2 out]
      }
      event "返回": Value Change {
        n193 = event-data() -> ()  [unwired: 1 in, 6 out]
        n194 = property on="窗格" class="Pane"("Origin"=T6 {"Horizontal"=0, "Vertical"=0} ("原点")) -> ()  [unwired: 2 in, 2 out]
      }
      event "标液浓度1", "测量吸光度1", "测量吸光度2", "标液浓度2", "测量吸光度3", "标液浓度3", "测量吸光度4", "标液浓度4", "测量吸光度5", "标液浓度5", "样品1启用", "样品3启用", "样品4启用", "样品5启用", "样品2启用", "模型", "method", "样品1 F0", "样品1 F1", "样品2 F1", "样品2 F0", "样品3 F1", "样品4 F0", "样品4 F1", "样品5 F1", "样品5 F0", "精度": Value Change {
        n195 = event-data() -> ()  [unwired: 1 in, 6 out]
        n196 = formula code="E=log(F0/F1);"("F0"="样品1 F0", "F1"="样品1 F1") -> ("E"=w393:dbl)
        "测量吸光度1" <- w393
        n197 = formula code="E=log(F0/F1);"("F0"="样品2 F0", "F1"="样品2 F1") -> ("E"=w390:dbl)
        "测量吸光度2" <- w390
        n198 = formula code="E=log(F0/F1);"("F0"="样品3 F0", "F1"="样品3 F1") -> ("E"=w387:dbl)
        "测量吸光度3" <- w387
        n199 = formula code="E=log(F0/F1);"("F0"="样品4 F0", "F1"="样品4 F1") -> ("E"=w384:dbl)
        "测量吸光度4" <- w384
        n200 = formula code="E=log(F0/F1);"("F0"="样品5 F0", "F1"="样品5 F1") -> ("E"=w381:dbl)
        "测量吸光度5" <- w381
        n201 = Replace Array Subset(array=dbl[] [0.0, 0.0, 0.0, 0.0, 0.0] ("数组"), new element #1="标液浓度1", new element #2="标液浓度2", new element #3="标液浓度3", new element #4="标液浓度4", new element #5="标液浓度5") -> (w378:dbl[])  [unwired: 5 in]
        n202 = Replace Array Subset(array=dbl[] [0.0, 0.0, 0.0, 0.0, 0.0] ("数组"), new element #1=w393, new element #2=w390, new element #3=w387, new element #4=w384, new element #5=w381) -> (w377:dbl[])  [unwired: 5 in]
        n203 = Replace Array Subset(array=bool[] [FALSE, FALSE, FALSE, FALSE, FALSE] ("数组"), new element #1="样品1启用", new element #2="样品2启用", new element #3="样品3启用", new element #4="样品4启用", new element #5="样品5启用") -> (w376:bool[])  [unwired: 5 in]
        n204 = call "线性公式.vi"("精度"="精度", "模型"="模型", "method"="method", "启用"=w376, "监测浓度"=w377, "标液浓度"=w378) -> ("XY图"=→"XY图":cluster{"X Values":dbl[], "Y Values":dbl[]}[], "r^2"=→"r^2":dbl, "拟合方程"=→"拟合公式":string)  [unwired: 3 in]
      }
      event "标液浓度1", "标液浓度2", "标液浓度3", "标液浓度4", "标液浓度5", "样品1 F0", "样品1 F1", "样品2 F1", "样品2 F0", "样品3 F1", "样品3 F0", "样品4 F0", "样品4 F1", "样品5 F0", "样品5 F1", "精度", "公式.X^2", "公式.X", "公式.b", "量程切换阈值.阈值", "量程切换阈值.标液浓度", "备用系数.量程上限", "备用系数.量程下限", "备用系数.检出限", "备用系数.精度": Mouse Down {
        n205 = event-data() -> ("CtlRef"=w412:refnum<vi>)  [unwired: 1 in, 5 out]
        n206 = property class="DigNum (严格)"(reference=w412) -> (reference out=w410:refnum<vi>, "Value"=w411:dbl)  [unwired: 1 in, 1 out]
        n207 = call "数字键盘.vi"("OldNumber"=w411) -> ("NewNumber"=w409:sgl)
        n208 = property class="DigNum (严格)"(reference=w410, "Val(Sgnl)"=w409) -> ()  [unwired: 1 in, 2 out]
      }
      event "读公式": Value Change {
        n209 = event-data() -> ()  [unwired: 1 in, 6 out]
        n210 = property class="Enum (严格)"(reference=w420) -> ("Value"=w419:enum16{"氨氮", "总磷"})  [unwired: 1 in, 2 out]
        n211 = property class="Enum (严格)"(reference=w421) -> ("Value"=w418:enum16{"水样测量", "空白核查", "标样核查", "盲样测试", "加标回收"})  [unwired: 1 in, 2 out]
        n212 = property class="Enum (严格)"(reference=w422) -> ("Value"=w417:enum16{"低量程", "高量程"})  [unwired: 1 in, 2 out]
        n213 = call "总磷氨氮公式读取.vi"("量程"=w417, "测量模式"=w418, "测量参数"=w419) -> ("error out"=w414:errorcluster, "公式"=w415:cluster{"X^2":dbl, "X":dbl, "b":dbl})  [unwired: 7 in]
        n214 = property class="Clust (严格)"(reference=w416, "Value"=w415) -> ()  [unwired: 1 in, 2 out]
        n215 = case shown="错误" w414 {
          tunnel: ["读取成功" ("消息") "读取失败" ("消息")] -> w413
          frame No Error {
          }
          frame Error {
          }
        }
        n216 = One Button Dialog(message=w413) -> ()  [unwired: 1 in, 1 out]
      }
      event "写公式": Value Change {
        n217 = event-data() -> ()  [unwired: 1 in, 6 out]
        n218 = call "总磷氨氮公式写入.vi"("公式"="公式", "量程"="量程下拉列表", "测量模式"="测量模式下拉列表", "测量参数"="参数下拉列表") -> ("error out"=w425:errorcluster)  [unwired: 7 in]
        n219 = case shown="无错误" w425 {
          tunnel: ["写入成功" ("消息") "写入失败" ("消息")] -> w426
          frame No Error {
          }
          frame Error {
          }
        }
        n220 = One Button Dialog(message=w426) -> ()  [unwired: 1 in, 1 out]
      }
      event "量程切换阈值读取": Value Change {
        n221 = event-data() -> ()  [unwired: 1 in, 6 out]
        n222 = property class="Enum (严格)"(reference=w440) -> ("Value"=w439:enum16{"氨氮", "总磷"})  [unwired: 1 in, 2 out]
        n223 = property class="Enum (严格)"(reference=w441) -> ("Value"=w438:enum16{"水样测量", "空白核查", "标样核查", "盲样测试", "加标回收"})  [unwired: 1 in, 2 out]
        n224 = property class="Enum (严格)"(reference=w442) -> ("Value"=w437:enum16{"低量程", "高量程"})  [unwired: 1 in, 2 out]
        n225 = call "总磷氨氮量程读取.vi"("量程"=w437, "测量模式"=w438, "测量参数"=w439) -> ("error out"=w433:errorcluster, "量程切换阈值"=w435:cluster{"阈值":dbl, "标液浓度":dbl})  [unwired: 7 in]
        n226 = property class="Clust (严格)"(reference=w436, "Value"=w435) -> ()  [unwired: 1 in, 2 out]
        n227 = case shown="错误" w433 {
          tunnel: ["读取成功" ("消息") "读取失败" ("消息")] -> w434
          frame No Error {
          }
          frame Error {
          }
        }
        n228 = One Button Dialog(message=w434) -> ()  [unwired: 1 in, 1 out]
      }
      event "量程切换阈值写入": Value Change {
        n229 = event-data() -> ()  [unwired: 1 in, 6 out]
        n230 = property class="Enum (严格)"(reference=w453) -> ("Value"=w450:enum16{"氨氮", "总磷"})  [unwired: 1 in, 2 out]
        n231 = property class="Enum (严格)"(reference=w452) -> ("Value"=w449:enum16{"水样测量", "空白核查", "标样核查", "盲样测试", "加标回收"})  [unwired: 1 in, 2 out]
        n232 = property class="Enum (严格)"(reference=w451) -> ("Value"=w448:enum16{"低量程", "高量程"})  [unwired: 1 in, 2 out]
        n233 = call "总磷氨氮量程写入.vi"("量程切换阈值"="量程切换阈值", "量程"=w448, "测量模式"=w449, "测量参数"=w450) -> ("error out"=w445:errorcluster)  [unwired: 7 in]
        n234 = case shown="无错误" w445 {
          tunnel: ["写入成功" ("消息") "写入失败" ("消息")] -> w446
          frame No Error {
          }
          frame Error {
          }
        }
        n235 = One Button Dialog(message=w446) -> ()  [unwired: 1 in, 1 out]
      }
      event "备用系数读取": Value Change {
        n236 = event-data() -> ()  [unwired: 1 in, 6 out]
        n237 = property class="Enum (严格)"(reference=w461) -> ("Value"=w460:enum16{"氨氮", "总磷"})  [unwired: 1 in, 2 out]
        n238 = call "总磷氨氮备用系数读取.vi"("测量参数"=w460) -> ("error out"=w456:errorcluster, "备用系数"=w458:T2)  [unwired: 9 in]
        n239 = property class="Clust (严格)"(reference=w459, "Value"=w458) -> ()  [unwired: 1 in, 2 out]
        n240 = case shown="错误" w456 {
          tunnel: ["读取成功" ("消息") "读取失败" ("消息")] -> w457
          frame No Error {
          }
          frame Error {
          }
        }
        n241 = One Button Dialog(message=w457) -> ()  [unwired: 1 in, 1 out]
      }
      event "备用系数写入": Value Change {
        n242 = event-data() -> ()  [unwired: 1 in, 6 out]
        n243 = property class="Enum (严格)"(reference=w468) -> ("Value"=w467:enum16{"氨氮", "总磷"})  [unwired: 1 in, 2 out]
        n244 = call "总磷氨氮备用系数写入.vi"("备用系数"="备用系数", "测量参数"=w467) -> ("error out"=w464:errorcluster)  [unwired: 9 in]
        n245 = case shown="无错误" w464 {
          tunnel: ["写入成功" ("消息") "写入失败" ("消息")] -> w465
          frame No Error {
          }
          frame Error {
          }
        }
        n246 = One Button Dialog(message=w465) -> ()  [unwired: 1 in, 1 out]
      }
    }
  }
  n247 = while {
    tunnel: w34 -> [w479]
    tunnel: w35 -> [_]
    shift-right: [w471] -> _
    shift-left: enum16{"氨氮", "总磷"}."氨氮" ("枚举") -> [w473]
    stop <- FALSE stop-if-true
    # "试剂填充 172 \n管路清洗108\n氨氮92\n总磷131\n总磷海水147\n总氮76\n总氮海水92"
    n248 = case shown="\"氨氮\", 默认" w473 {
      selector: w473 -> [w485 w487]
      tunnel: [w486 w488] -> w474
      tunnel: [w485 w487] -> w472
      frame "氨氮", Default {
        w486 = u16 3 items=["总磷"=1, "氨氮"=3] ("站号")
      }
      frame "总磷" {
        w488 = u16 1 items=["总磷"=1, "氨氮"=3] ("站号")
      }
    }
    n249 = Wait (ms)(milliseconds to wait=u32 1000 ("等待时间（毫秒）")) -> ()  [unwired: 1 out]
    n250 = Bundle By Name(cluster=cluster{"命令":string, "data":variant} {"命令"="", "data"=variant} ("元素"), "命令"="读状态告警区", "data"=w474) -> (w481:cluster{"命令":string, "data":variant})
    n251 = Enqueue Element(queue=w479, element=w481) -> (queue out=w475:refnum<queue>)  [unwired: 2 in, 2 out]
    n252 = Increment(x=w472) -> (x+1=w471:enum16{"氨氮", "总磷"})
    n253 = Bundle By Name(cluster=cluster{"命令":string, "data":variant} {"命令"="", "data"=variant} ("元素"), "命令"="读测量数据区", "data"=w474) -> (w477:cluster{"命令":string, "data":variant})
    n254 = Enqueue Element(queue=w475, element=w477) -> ()  [unwired: 2 in, 3 out]
  }
  n255 = Open VI Reference(type specifier VI Refnum (for type only)=refnum<vi> refnum, vi path=w30, options=128 ("选项")) -> (vi reference=w28:refnum<vi>, error out=w26:errorcluster)  [unwired: 3 in]
  n256 = call-by-ref "?"(reference=w28, error in=w26) -> (reference out=w24:refnum<vi>, error out=w25:errorcluster)  [unwired: 12 in]
  n257 = Open VI Reference(type specifier VI Refnum (for type only)=refnum<vi> refnum, vi path=w16, options=128 ("选项")) -> (vi reference=w18:refnum<vi>, error out=w20:errorcluster)  [unwired: 3 in]
  n258 = call-by-ref "?"(reference=w18, error in=w20) -> (reference out=w22:refnum<vi>, error out=w21:errorcluster)  [unwired: 12 in]
  n259 = Close Reference(reference=w24, error in (no error)=w25) -> ()  [unwired: 1 out]
  n260 = Close Reference(reference=w22, error in (no error)=w21) -> ()  [unwired: 1 out]
  n261 = node-c288(w4) -> ()  [unwired: 1 out]
